vi "Update Waveform to Graph.vi"(8 "Stop Channel":T1, 9 "Scope Recording Settings":T2 {"Fetch Timeout" format="%.2f"}, 10 "Waveform Channel":T3, 11 "WaveformGraph Ref":refnum<class "Live Graph Plotter.lvclass">) -> (0 "error out":errorcluster)   [LabVIEW 2025]
uses:
  Live Graph Plotter/Live Graph Plotter.lvclass
  <extravilib>/ChannelInstances/Stream-a[.](c(dbl,dbl,a[.](dbl))).lvlib
  <extravilib>/ChannelInstances/Tag-bool.lvlib
  <extravilib>/ChannelInstances/Stream-a[.](c(dbl,dbl,a[.](dbl)))/)Channel.ctl
  Typedef/Scope Recording Settings.ctl
  <extravilib>/ChannelInstances/Tag-bool/))Channel.ctl
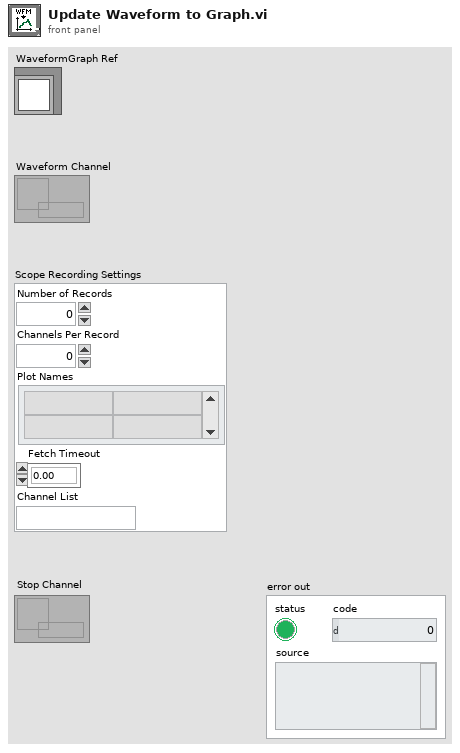
[diagram p1: front panel]
types:
  T1 = typedef "Tag-bool.lvlib/))Channel.ctl" = refnum<queue>
  T2 = typedef "Scope Recording Settings.ctl" = cluster{"Number of Records":i32, "Channels Per Record":i32, "Plot Names":string[][], "Fetch Timeout":dbl, "Channel List":string}
  T3 = typedef "Stream-a[.](c(dbl,dbl,a[.](dbl))).lvlib/)Channel.ctl" = refnum<queue>
  T4 = cluster{"relativeInitialX":dbl, "xIncrement":dbl, "wfm":dbl[]}[]
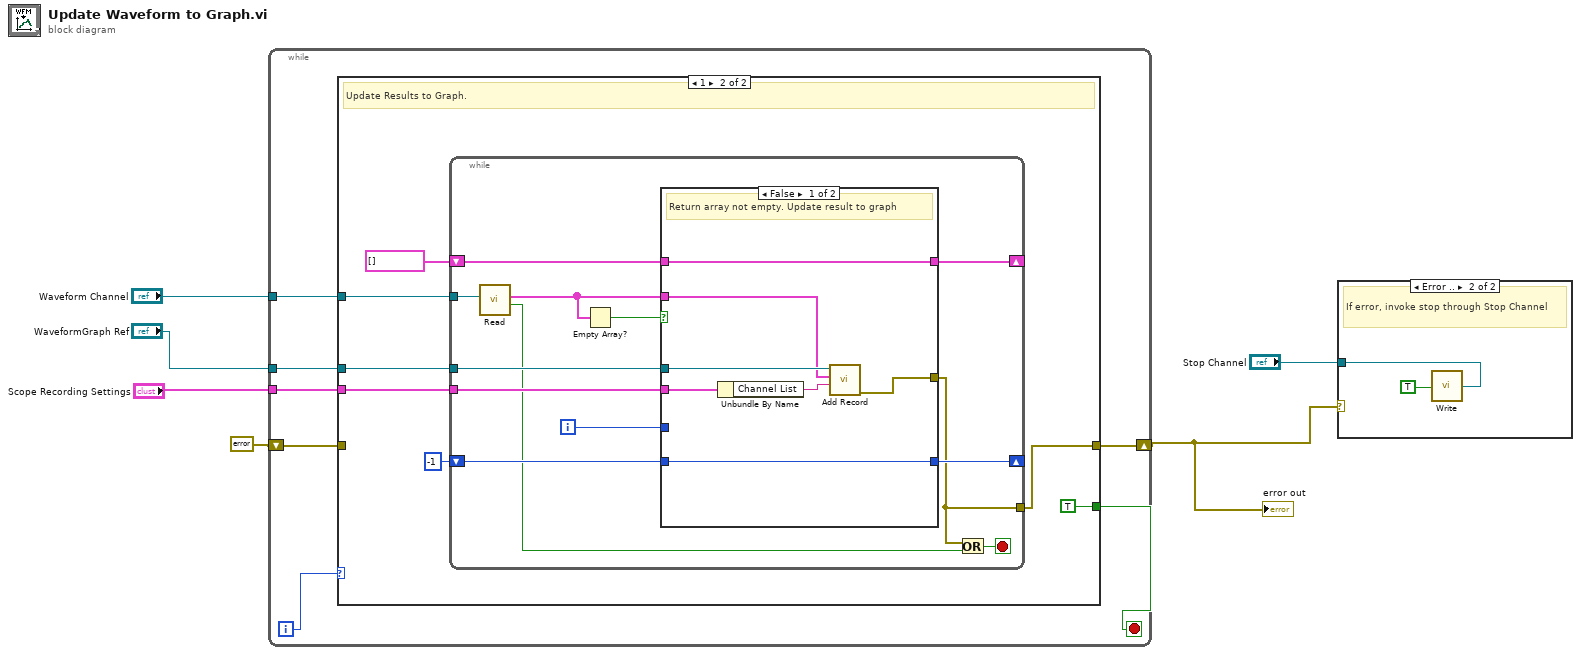
[diagram p0: block diagram]
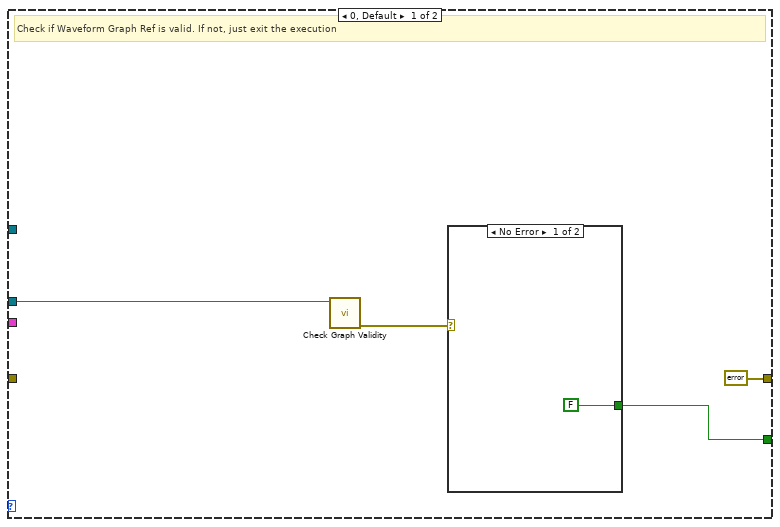
[diagram p2: hidden frame]
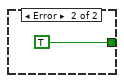
[diagram p3: hidden frame]
diagram:
  n1 = while {
    tunnel: "Waveform Channel" -> [w13]
    tunnel: "Scope Recording Settings" -> [w12]
    tunnel: "WaveformGraph Ref" -> [w11]
    shift-right: [w8] -> w1
    shift-left: errorcluster {"status"=FALSE, "code"=0, "source"=""} ("error out") -> [w7]
    i -> [w10]
    stop <- w9 stop-if-true
    n2 = case shown="1" w10 {
      tunnel: w13 -> [_ w25]
      tunnel: w12 -> [_ w24]
      tunnel: w11 -> [w14 w23]
      tunnel: [w16 TRUE ("f")] -> w9
      tunnel: [errorcluster {"status"=FALSE, "code"=0, "source"=""} ("error out") w21] -> w8
      tunnel: w7 -> [_ _]
      frame 0, Default {
        # "Check if Waveform Graph Ref is valid. If not, just exit the execution"
        n3 = call "Check Graph Validity.vi"("Live Graph Plotter in"=w14) -> ("error out"=w17:errorcluster)  [unwired: 9 in, 1 out]
        n4 = case shown="No Error" w17 {
          tunnel: [FALSE TRUE] -> w16
          frame No Error {
          }
          frame Error {
          }
        }
      }
      frame 1 {
        # "Update Results to Graph."
        n5 = while {
          tunnel: w24 -> [w30]
          tunnel: w23 -> [w39]
          tunnel: w25 -> [w38]
          shift-right: [w36] -> _
          shift-left: T4 [] -> [w37]
          shift-right: [w34] -> _
          shift-left: -1 -> [w35]
          tunnel: [w27] -> w21
          i -> [w32]
          stop <- w28 stop-if-true
          n6 = call <extravilib>:"Read.vi"("channel"=w38) -> ("last element?"=w29:bool, "element"=w33:T4)  [unwired: 6 in, 3 out]
          n7 = Empty Array?(array=w33) -> (empty?=w31:bool)
          n8 = case shown="False" w31 {
            tunnel: w39 -> [w46 _]
            tunnel: w37 -> [w45 w47]
            tunnel: [w45 w47] -> w36
            tunnel: w35 -> [w44 w48]
            tunnel: [w44 w48] -> w34
            tunnel: w33 -> [w43 _]
            tunnel: w32 -> [_ _]
            tunnel: w30 -> [w42 _]
            tunnel: [w41 _] -> w27
            frame False {
              # "Return array not empty. Update result to graph"
              n9 = Unbundle By Name(w42) -> ("Channel List"=w40:string)
              n10 = call "Add Record.vi"("Channel List"=w40, "Waveforms"=w43, "Live Graph Plotter in"=w46) -> ("error out"=w41:errorcluster)  [unwired: 7 in, 1 out]
            }
            frame True {
              # "Result is empty array. Skip the plot index"
            }
          }
          n11 = Or(x=w27, y=w29) -> (x .or. y?=w28:bool)
        }
      }
    }
  }
  "error out" <- w1
  n12 = case shown="Error .." w1 {
    tunnel: "Stop Channel" -> [_ w49]
    frame No Error {
    }
    frame Error {
      # "If error, invoke stop through Stop Channel"
      n13 = call <extravilib>:"Write.vi"("element"=TRUE) -> ("channel"=w49:T1)  [unwired: 1 out]
    }
  }
